vi "Cascade Logic Stub.vi"() -> ()   [LabVIEW 2011]
uses:
  <vilib>/rvi/DataTransferAndStorage/Container/XNode/niFpgaContainer.xnode
  <vilib>/rvi/Memory/Memory_Emulation/niFpgaMemoryEmulationDramRetrieveDataRefIn.vi
panel:
  out "RetrieveData2_Next":bool
  out "RetrieveData1_Next":bool
  out "UsePrev1_Next":bool
  out "UsePrev1_Next":bool
  out "Datavalid2_Out":bool
  out "DataValid1_Out":bool
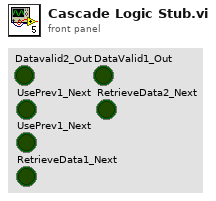
[diagram p1: front panel]
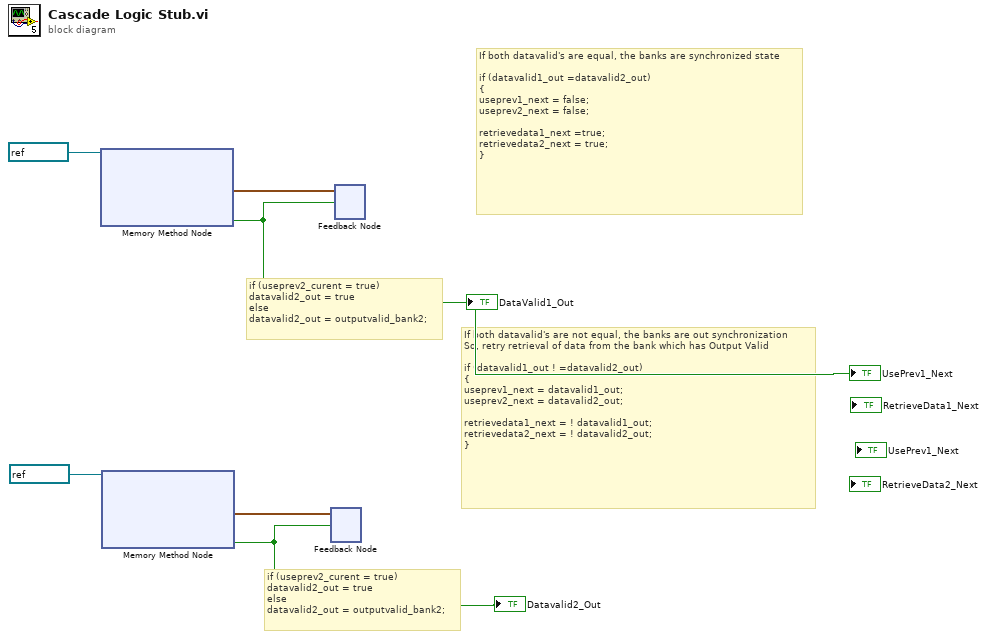
[diagram p0: block diagram]
diagram:
  # "if (useprev2_curent = true)\ndatavalid2_out = true\nelse\ndatavalid2_out = outputvalid_bank2;"
  # "If both datavalid's are equal, the banks are synchronized state\n\nif (datavalid1_out =datavalid2_out)\n{\nuseprev1_next = false;\nuseprev2_next = false;\n\nretrievedata1_next =true;\nretrievedata2_next = true;\n}"
  # "if (useprev2_curent = true)\ndatavalid2_out = true\nelse\ndatavalid2_out = outputvalid_bank2;"
  # "If both datavalid's are not equal, the banks are out synchronization\nSo, retry retrieval of data from the bank which has Output Valid\n\nif (datavalid1_out ! =datavalid2_out)\n{\nuseprev1_next = datavalid1_out;\nuseprev2_next = datavalid2_out;\n\nretrievedata1_next = ! datavalid1_out;\nretrievedata2_next = ! datavalid2_out;\n}"
  n1 = xnode ("Memory Method Node")("Memory In"=refnum<k21> "Bank0") -> ("Data"=w5:cluster{"high":u64, "low":u64}, "Output Valid"=w1:bool)  [unwired: 1 in, 1 out]
  "DataValid1_Out" <- w1
  "UsePrev1_Next" <- w1
  n2 = xnode ("Memory Method Node")("Memory In"=refnum<k21> "Bank0") -> ("Data"=w3:cluster{"high":u64, "low":u64}, "Output Valid"=w2:bool)  [unwired: 1 in, 1 out]
  "Datavalid2_Out" <- w2
  n3 = feedback #1() -> ()  [unwired: 2 in]
  n4 = feedback-in #1(w3, w2) -> ()
  n5 = feedback #2() -> ()  [unwired: 2 in]
  n6 = feedback-in #2(w5, w1) -> ()
